vi "autopilot.vi"() -> ()   [LabVIEW 2016]
uses:
  <vilib>/LVH/AR Drone Toolkit/Decode NavData/Typedefs/NavData Demo.ctl
  <vilib>/LVH/AR Drone Toolkit/AR Drone.lvlib
panel:
  out "NavData Out":T1
  out "11":bool
  out "10":bool
  out "9":bool
  out "12":bool
  out "8":bool
  out "7":bool
  out "6":bool
  out "5":bool
  out "4":bool
  out "3":bool
  out "2":bool
  out "1":bool
  out "error out":errorcluster
  out "close_conn":bool
  out "autopilot?":bool
  out "Video Stream":picture
  out "battery percentage":u32(knob) scale=0.0..100.0
  out "pitch_speed":dbl
  out "roll_speed":dbl
  out "Hovering?":bool
  out "active_height_correction":bool
  out "active_yaw_correction":bool
  out "set_height?":bool
  out "height_speed":sgl
  out "set_height":i32
  out "set_yaw?":bool
  out "yaw_speed":sgl
  out "set_yaw":dbl
  in  "start":bool
  in  "Nr photos":i32
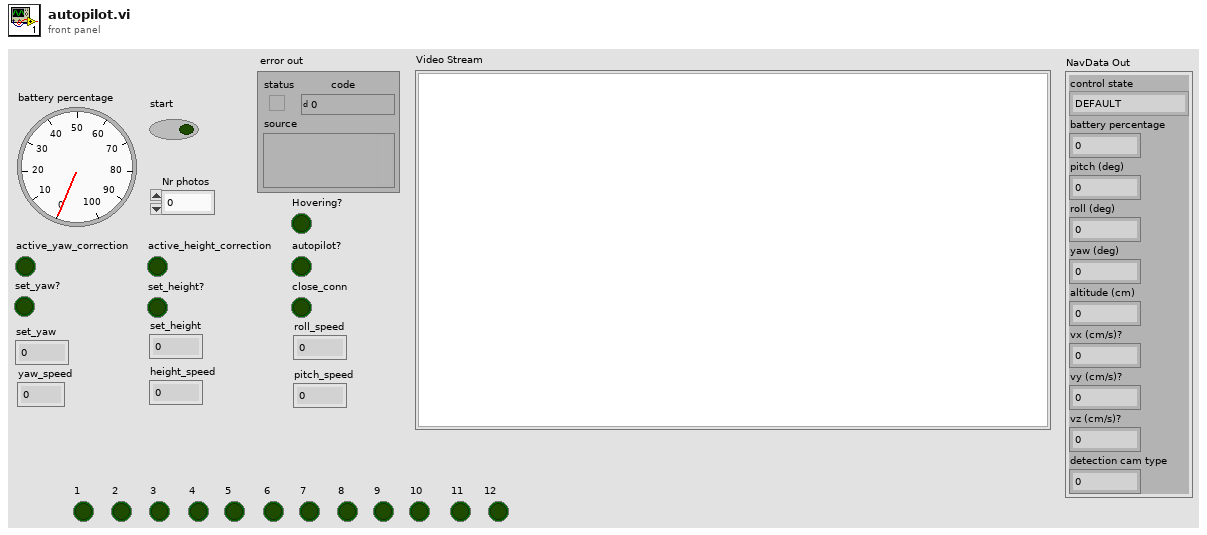
[diagram p1: front panel]
types:
  T1 = typedef "AR Drone.lvlib/NavData Demo.ctl" = cluster{"control state":enum32{"DEFAULT", "INIT", "LANDING", "FLYING", "HOVERING", "TEST", "TRANS_TAKEOFF", "TRANS_GOTOFIX", "TRANS_LANDING"}, "battery percentage":u32, "pitch (deg)":sgl, "roll (deg)":sgl, "yaw (deg)":sgl, "altitude (cm)":u32, "vx (cm/s)?":sgl, "vy (cm/s)?":sgl, "vz (cm/s)?":sgl, "detection cam type":u32}
  T2 = cluster{"Drone IP address":string, "Home IP address":string, "Flight Mode":enum8{"OUTDOOR MODE", "INDOOR MODE"}, "Mounted Hull":enum8{"OUTDOOR HULL", "INDOOR HULL"}, "Video Camera":u8, "Max Altitude (m)":sgl, "Max Pitch and Roll Angle (deg)":sgl, "Max Vertical Speed (m/s)":sgl, "Max Yaw Speed (deg/s)":sgl}
  T3 = typedef "AR Drone.lvlib/AR Drone Resource.ctl" = cluster{"UDP Control Connection":refnum<k16>, "UDP NavData Connection":refnum<k16>, "UDP Video Connection (Drone 1.0)":refnum<k16>, "TCP Video Connection (Drone 2.0)":refnum<k5>, "TCP Control Port Connection":refnum<k5>, "Drone IP address":string, "Drone Command Port":u16, "Drone NavData Port":u16, "Drone Vid Stream Port":u16, "Drone TCP Control Port":u16, "Home IP address":string, "Home Command Port":u16, "Home NavData Port":u16, "Home Vid Stream Port":u16, "Drone Version":i32, "Drone Index":i32, "Command Sequence":i32}
  T4 = cluster{"Roll":sgl, "Pitch":sgl, "height_speed":sgl, "yaw_speed":sgl}
  T5 = cluster{"roll_speed":dbl, "pitch_speed":dbl, "height_speed":sgl, "yaw_speed":sgl}
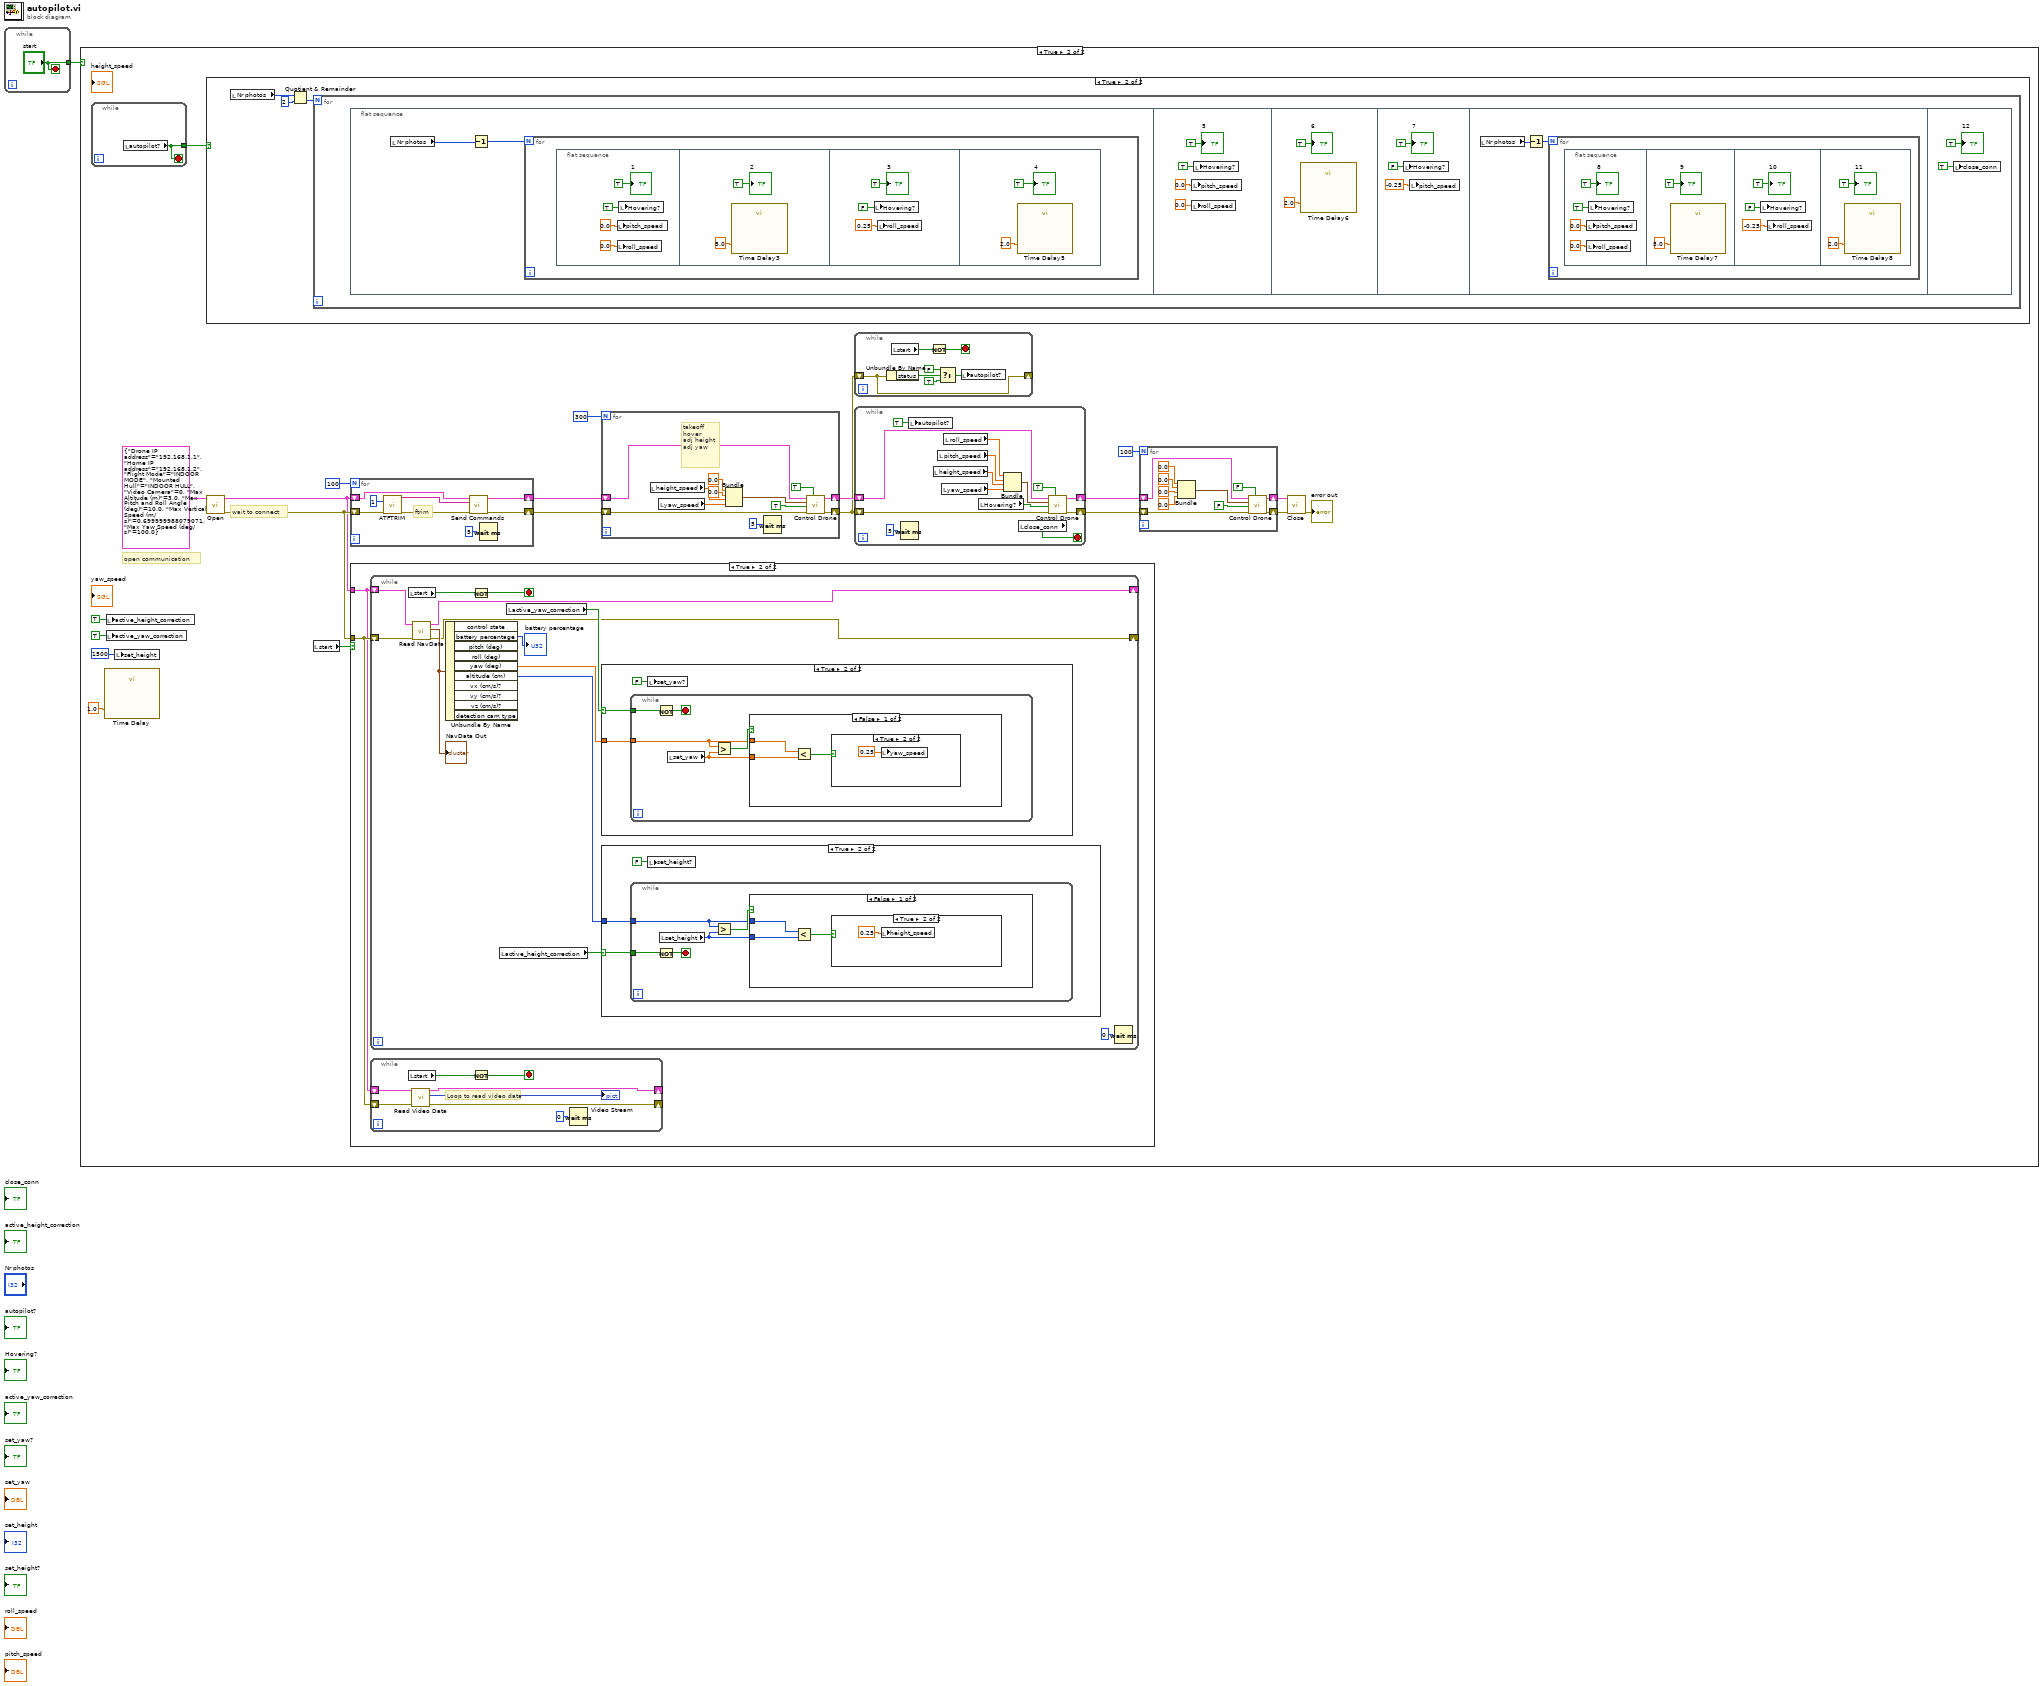
[diagram p0: block diagram]
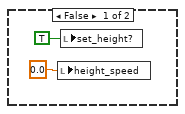
[diagram p4: hidden frame]
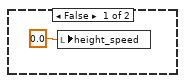
[diagram p5: hidden frame]
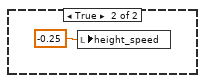
[diagram p6: hidden frame]
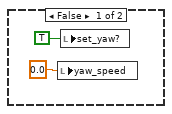
[diagram p7: hidden frame]
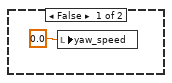
[diagram p8: hidden frame]
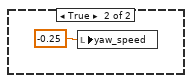
[diagram p9: hidden frame]
diagram:
  n1 = while {
    tunnel: ["start"] -> w1
    stop <- "start" stop-if-true
  }
  n2 = case shown="True" w1 {
    frame False {
    }
    frame True {
      # "wait to connect"
      # "open communication"
      n3 = while {
        tunnel: [w35] -> w23
        stop <- w35 stop-if-true
        n4 = local read "autopilot?"() -> (w35:bool)
      }
      n5 = call "Time Delay"("Delay Time (s)"=1.0) -> ()  [unwired: 10 in, 1 out]
      n6 = local write "active_height_correction"(TRUE) -> ()
      n7 = local write "active_yaw_correction"(TRUE) -> ()
      n8 = local write "set_height"(1500 ("set_height")) -> ()
      n9 = case shown="True" w23 {
        frame False {
        }
        frame True {
          n10 = local read "Nr photos"() -> (w134:i32)
          n11 = Quotient & Remainder(x=w134, y=2) -> (floor(x/y)=w132:i32)  [unwired: 1 out]
          n12 = for {
            N: w132 -> [_]
            n13 = flat-sequence {
              frame #0 {
                n14 = local read "Nr photos"() -> (w135:i32)
                n15 = Decrement(x=w135) -> (x-1=w136:i32)
                n16 = for {
                  N: w136 -> [_]
                  n17 = flat-sequence {
                    frame #0 {
                      n18 = local write "pitch_speed"(0.0 ("pitch_speed")) -> ()
                      n19 = local write "roll_speed"(0.0 ("roll_speed")) -> ()
                      n20 = local write "Hovering?"(TRUE) -> ()
                      "1" <- TRUE ("1")
                    }
                    frame #1 {
                      n21 = call "Time Delay3"("Delay Time (s)"=5.0) -> ()  [unwired: 10 in, 1 out]
                      "2" <- TRUE ("2")
                    }
                    frame #2 {
                      n22 = local write "Hovering?"(FALSE) -> ()
                      n23 = local write "roll_speed"(0.25 ("roll_speed")) -> ()
                      "3" <- TRUE ("3")
                    }
                    frame #3 {
                      n24 = call "Time Delay5"("Delay Time (s)"=2.0) -> ()  [unwired: 10 in, 1 out]
                      "4" <- TRUE ("4")
                    }
                  }
                }
              }
              frame #1 {
                n25 = local write "pitch_speed"(0.0 ("pitch_speed")) -> ()
                n26 = local write "roll_speed"(0.0 ("roll_speed")) -> ()
                n27 = local write "Hovering?"(TRUE) -> ()
                "5" <- TRUE ("5")
              }
              frame #2 {
                n28 = call "Time Delay6"("Delay Time (s)"=2.0) -> ()  [unwired: 10 in, 1 out]
                "6" <- TRUE ("6")
              }
              frame #3 {
                n29 = local write "Hovering?"(FALSE) -> ()
                n30 = local write "pitch_speed"(-0.25 ("pitch_speed")) -> ()
                "7" <- TRUE ("7")
              }
              frame #4 {
                n31 = local read "Nr photos"() -> (w157:i32)
                n32 = Decrement(x=w157) -> (x-1=w158:i32)
                n33 = for {
                  N: w158 -> [_]
                  n34 = flat-sequence {
                    frame #0 {
                      n35 = local write "pitch_speed"(0.0 ("pitch_speed")) -> ()
                      n36 = local write "roll_speed"(0.0 ("roll_speed")) -> ()
                      n37 = local write "Hovering?"(TRUE) -> ()
                      "8" <- TRUE ("8")
                    }
                    frame #1 {
                      n38 = call "Time Delay7"("Delay Time (s)"=5.0) -> ()  [unwired: 10 in, 1 out]
                      "9" <- TRUE ("9")
                    }
                    frame #2 {
                      n39 = local write "Hovering?"(FALSE) -> ()
                      n40 = local write "roll_speed"(-0.25 ("roll_speed")) -> ()
                      "10" <- TRUE ("10")
                    }
                    frame #3 {
                      n41 = call "Time Delay8"("Delay Time (s)"=2.0) -> ()  [unwired: 10 in, 1 out]
                      "11" <- TRUE ("11")
                    }
                  }
                }
              }
              frame #5 {
                n42 = local write "close_conn"(TRUE) -> ()
                "12" <- TRUE ("12")
              }
            }
          }
        }
      }
      n43 = call <vilib>:"Open.vi"("Setup Parameters"=T2 {"Drone IP address"="192.168.1.1", "Home IP address"="192.168.1.2", "Flight Mode"=enum."INDOOR MODE", "Mounted Hull"=enum."INDOOR HULL", "Video Camera"=0, "Max Altitude (m)"=3.0, "Max Pitch and Roll Angle (deg)"=10.0, "Max Vertical Speed (m/s)"=0.7, "Max Yaw Speed (deg/s)"=100.0}) -> ("error out"=w22:errorcluster, "AR Drone Resource"=w21:T3)  [unwired: 9 in]
      n44 = local read "start"() -> (w16:bool)
      n45 = for {
        N: 100 -> [_]
        shift-right: [w64] -> w18
        shift-left: w21 -> [w66]
        shift-right: [w63] -> w17
        shift-left: w22 -> [w65]
        # "ftrim"
        n46 = call <vilib>:"ATFTRIM.vi"("Command Sequence"=1, "error in (no error)"=w65) -> ("Command String out"=w67:string, "error out"=w68:errorcluster)  [unwired: 11 in, 1 out]
        n47 = call <vilib>:"Send Commands.vi"("error in (no error)"=w68, "Command String"=w67, "AR Drone Resource"=w66) -> ("error out"=w63:errorcluster, "AR Drone Resource Out"=w64:T3)  [unwired: 5 in]
        n48 = Wait (ms)(milliseconds to wait=u32 5) -> ()  [unwired: 1 out]
      }
      n49 = case shown="True" w16 {
        tunnel: w21 -> [_ w70]
        tunnel: w22 -> [_ w71]
        frame False {
        }
        frame True {
          n50 = while {
            shift-right: [w81] -> _
            shift-left: w70 -> [w82]
            shift-right: [w80] -> _
            shift-left: w71 -> [w83]
            stop <- w88 stop-if-true
            n51 = local read "start"() -> (w87:bool)
            n52 = call <vilib>:"Read NavData.vi"("error in (no error)"=w83, "AR Drone Resource"=w82) -> ("error out"=w80:errorcluster, "NavData Out"=w84:T1, "AR Drone Resource Out"=w81:T3)  [unwired: 7 in]
            "NavData Out" <- w84
            n53 = Unbundle By Name(w84) -> ("battery percentage"=→"battery percentage":u32, "yaw (deg)"=w89:sgl, "altitude (cm)"=w90:u32)  [unwired: 7 out]
            n54 = Not(x=w87) -> (.not. x?=w88:bool)
            n55 = local read "active_height_correction"() -> (w92:bool)
            n56 = local read "active_yaw_correction"() -> (w91:bool)
            n57 = case shown="True" w91 {
              selector: w91 -> [_ w113]
              tunnel: w89 -> [_ w112]
              frame False {
                n58 = local write "yaw_speed"(sgl 0.0) -> ()
                n59 = local write "set_yaw?"(TRUE) -> ()
              }
              frame True {
                n60 = while {
                  tunnel: w113 -> [w118]
                  tunnel: w112 -> [w114]
                  stop <- w117 stop-if-true
                  n61 = Not(x=w118) -> (.not. x?=w117:bool)
                  n62 = local read "set_yaw"() -> (w115:dbl)
                  n63 = Greater?(x=w114, y=w115) -> (0:w116:bool)
                  n64 = case shown="False" w116 {
                    tunnel: w115 -> [w121 _]
                    tunnel: w114 -> [w119 _]
                    frame False {
                      n65 = Less?(x=w119, y=w121) -> (x < y?=w120:bool)
                      n66 = case shown="True" w120 {
                        frame False {
                          n67 = local write "yaw_speed"(sgl 0.0) -> ()
                        }
                        frame True {
                          n68 = local write "yaw_speed"(sgl 0.25) -> ()
                        }
                      }
                    }
                    frame True {
                      n69 = local write "yaw_speed"(sgl -0.25) -> ()
                    }
                  }
                }
                n70 = local write "set_yaw?"(FALSE) -> ()
              }
            }
            n71 = case shown="True" w92 {
              selector: w92 -> [_ w97]
              tunnel: w90 -> [_ w96]
              frame False {
                n72 = local write "height_speed"(sgl 0.0) -> ()
                n73 = local write "set_height?"(TRUE) -> ()
              }
              frame True {
                n74 = while {
                  tunnel: w97 -> [w102]
                  tunnel: w96 -> [w98]
                  stop <- w101 stop-if-true
                  n75 = Not(x=w102) -> (.not. x?=w101:bool)
                  n76 = local read "set_height"() -> (w99:i32)
                  n77 = Greater?(x=w98, y=w99) -> (0:w100:bool)
                  n78 = case shown="False" w100 {
                    tunnel: w99 -> [w105 _]
                    tunnel: w98 -> [w103 _]
                    frame False {
                      n79 = Less?(x=w103, y=w105) -> (x < y?=w104:bool)
                      n80 = case shown="True" w104 {
                        frame False {
                          n81 = local write "height_speed"(sgl 0.0) -> ()
                        }
                        frame True {
                          n82 = local write "height_speed"(sgl 0.25) -> ()
                        }
                      }
                    }
                    frame True {
                      n83 = local write "height_speed"(sgl -0.25) -> ()
                    }
                  }
                }
                n84 = local write "set_height?"(FALSE) -> ()
              }
            }
            n85 = Wait (ms)(milliseconds to wait=u32 0) -> ()  [unwired: 1 out]
          }
          n86 = while {
            shift-right: [w72] -> _
            shift-left: w70 -> [w75]
            shift-right: [w79] -> _
            shift-left: w71 -> [w74]
            stop <- w77 stop-if-true
            # "Loop to read video data"
            n87 = local read "start"() -> (w76:bool)
            n88 = call <vilib>:"Read Video Data.vi"("error in (no error)"=w74, "AR Drone Resource"=w75) -> ("error out"=w79:errorcluster, "Video Stream"=→"Video Stream":picture, "AR Drone Resource Out"=w72:T3)  [unwired: 7 in]
            n89 = Not(x=w76) -> (.not. x?=w77:bool)
            n90 = Wait (ms)(milliseconds to wait=u32 0) -> ()  [unwired: 1 out]
          }
        }
      }
      n91 = for {
        N: 300 -> [_]
        shift-right: [w54] -> w20
        shift-left: w18 -> [w56]
        shift-right: [w53] -> w19
        shift-left: w17 -> [w55]
        # "takeoff\nhover\nadj height\nadj yaw"
        n92 = local read "height_speed"() -> (w51:sgl)
        n93 = local read "yaw_speed"() -> (w50:sgl)
        n94 = Bundle("Roll"=sgl 0.0, "Pitch"=sgl 0.0, "height_speed"=w51, "yaw_speed"=w50) -> (w57:T4)  [unwired: 1 in]
        n95 = Wait (ms)(milliseconds to wait=u32 5) -> ()  [unwired: 1 out]
        n96 = call <vilib>:"Control Drone.vi"("Takeoff/Land"=TRUE, "error in (no error)"=w55, "Hover"=TRUE, "Control Cluster"=w57, "AR Drone Resource"=w56) -> ("error out"=w53:errorcluster, "AR Drone Resource Out"=w54:T3)  [unwired: 5 in]
      }
      n97 = while {
        shift-right: [w125] -> _
        shift-left: w19 -> [w125]
        stop <- w126 stop-if-true
        n98 = Unbundle By Name(w125) -> ("status"=w128:bool)
        n99 = local read "start"() -> (w127:bool)
        n100 = Not(x=w127) -> (.not. x?=w126:bool)
        n101 = Select(t=FALSE, s=w128, f=TRUE) -> (s? t:f=w129:bool)
        n102 = local write "autopilot?"(w129) -> ()
      }
      n103 = while {
        shift-right: [w39] -> w6
        shift-left: w20 -> [w47]
        shift-right: [w40] -> w5
        shift-left: w19 -> [w46]
        stop <- w38 stop-if-true
        n104 = Wait (ms)(milliseconds to wait=u32 5) -> ()  [unwired: 1 out]
        n105 = local write "autopilot?"(TRUE) -> ()
        n106 = local read "height_speed"() -> (w43:sgl)
        n107 = local read "pitch_speed"() -> (w41:dbl)
        n108 = local read "yaw_speed"() -> (w44:sgl)
        n109 = local read "roll_speed"() -> (w42:dbl)
        n110 = local read "Hovering?"() -> (w45:bool)
        n111 = Bundle("roll_speed"=w42, "pitch_speed"=w41, "height_speed"=w43, "yaw_speed"=w44) -> (w48:T5)  [unwired: 1 in]
        n112 = local read "close_conn"() -> (w38:bool)
        n113 = call <vilib>:"Control Drone.vi"("Takeoff/Land"=TRUE, "error in (no error)"=w46, "Hover"=w45, "Control Cluster"=w48, "AR Drone Resource"=w47) -> ("error out"=w40:errorcluster, "AR Drone Resource Out"=w39:T3)  [unwired: 5 in]
      }
      n114 = for {
        N: 100 -> [_]
        shift-right: [w24] -> w3
        shift-left: w6 -> [w27]
        shift-right: [w25] -> w4
        shift-left: w5 -> [w26]
        n115 = Bundle(sgl 0.0, sgl 0.0, sgl 0.0, sgl 0.0) -> (w34:cluster{sgl, sgl, sgl, sgl})  [unwired: 1 in]
        n116 = call <vilib>:"Control Drone.vi"("Takeoff/Land"=FALSE, "error in (no error)"=w26, "Hover"=FALSE, "Control Cluster"=w34, "AR Drone Resource"=w27) -> ("error out"=w25:errorcluster, "AR Drone Resource Out"=w24:T3)  [unwired: 5 in]
      }
      n117 = call <vilib>:"Close.vi"("error in (no error)"=w4, "AR Drone Resource"=w3) -> ("error out"=→"error out":errorcluster)  [unwired: 9 in]
    }
  }
